vi "Get Monitor Variables.vi"(8 "error in (no error)":errorcluster, 9 "Channel":i32, 11 "LabVIEW Web Service Request":refnum<class "Web Request.lvclass">) -> (0 "error out":errorcluster, 3 "LabVIEW Web Service Request out":refnum<class "Web Request.lvclass">)   [LabVIEW 2018]
doc: "This VI sets all of the ESP variables for a single contact so it can be output from an ESP script."
uses:
  <vilib>/wsapi/Web Request.lvclass
  subvis/i32 to dec string small.vi
  CAEN globals.vi
  <vilib>/wsapi/class/subVIs/Set Many String ESP Variables.vi
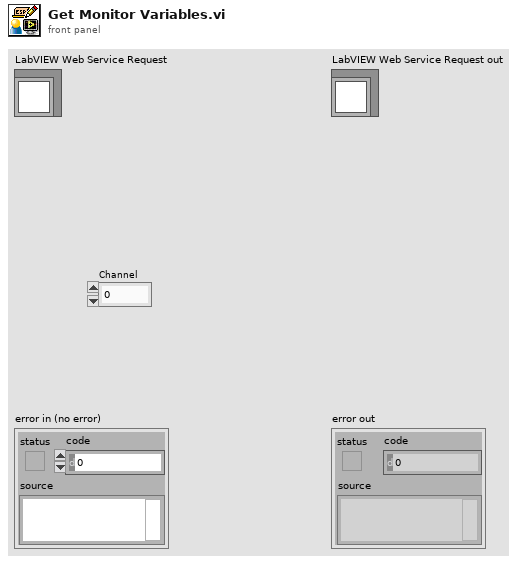
[diagram p1: front panel]
types:
  T1 = typedef "channel_cluster.ctl" = cluster{"Channel Name":string, "Crate":i32, "Card Type":string, "Card":i32, "Channel":i32, "Status Icon":picture, "Vmon (V)":dbl, "Vset (V)":dbl, "Imon (A)":dbl, "Iset (A)":dbl, "Timestamp":string, "ON/OFF":bool, "Status":string, "Vswmax (V)":dbl, "Flag":bool, "Vfile (V)":dbl, "Error Logged":bool[], "enable_file":bool}
  T2 = typedef "channel.ctl" = cluster{" Card.Channel":dbl, "Crate":i32}
  T3 = cluster{"Group Name":string, "Channels in Group":T2[]}[]
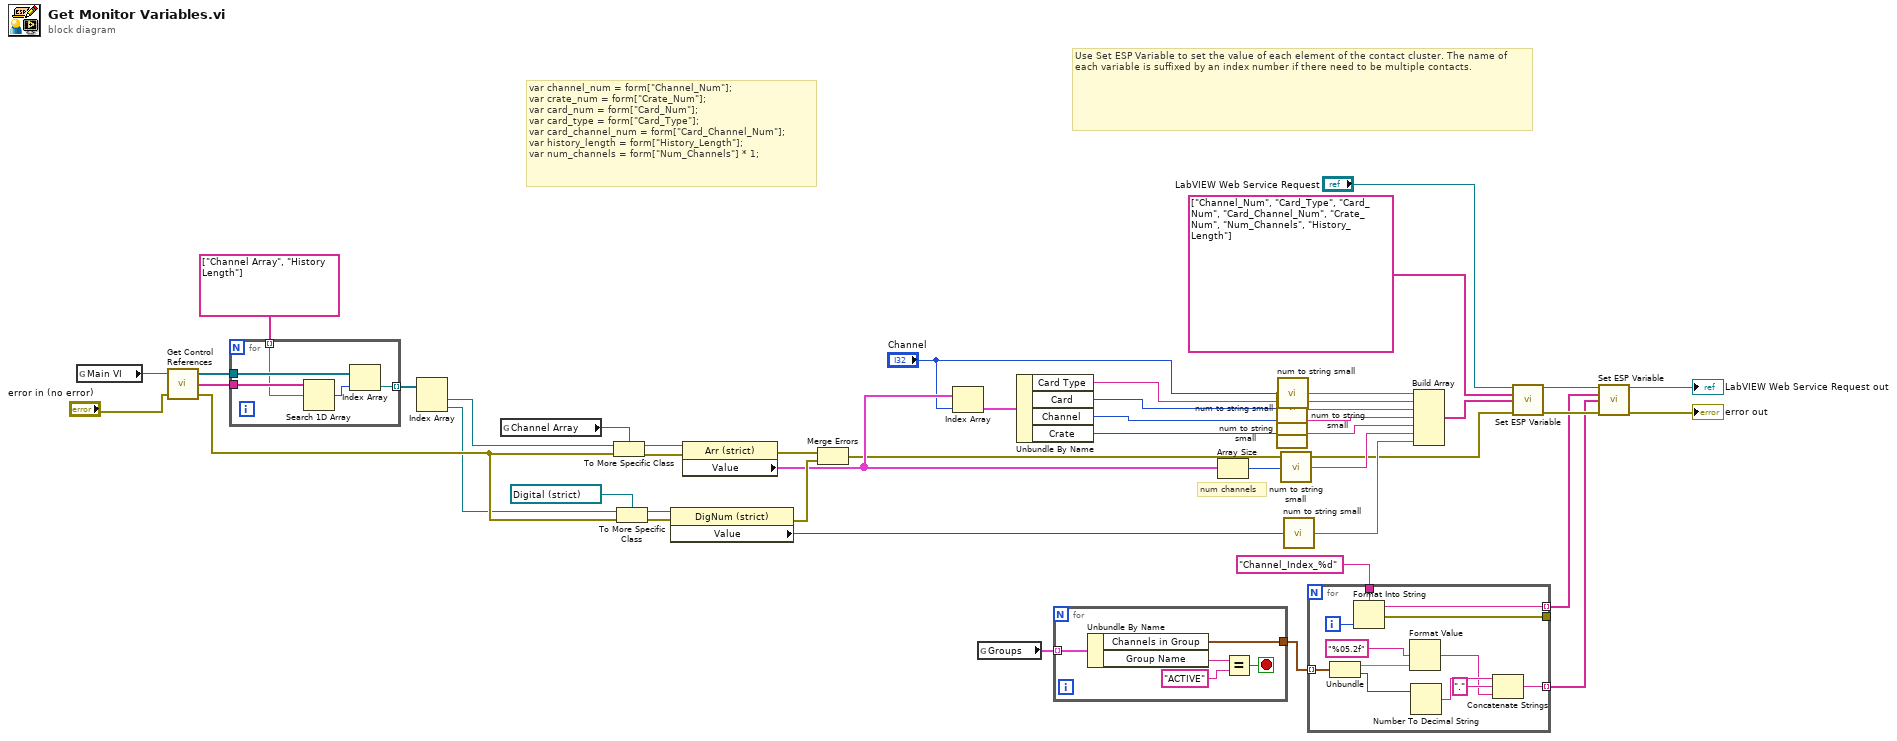
[diagram p0: block diagram]
diagram:
  # "var channel_num = form[\"Channel_Num\"]; \nvar crate_num = form[\"Crate_Num\"];\nvar card_num = form[\"Card_Num\"];\nvar card_type = form[\"Card_Type\"];\nvar card_channel_num = form[\"Card_Channel_Num\"];\nvar history_length = form[\"History_Length\"];\nvar num_channels = form[\"Num_Channels\"] * 1;"
  # "num channels"
  # "Use Set ESP Variable to set the value of each element of the contact cluster. The name of each variable is suffixed by an index number if there need to be multiple contacts."
  n1 = global read "CAEN globals.vi" "Main VI"() -> (w45:refnum<vi>)
  n2 = call "Get Control References.vi"("error in"="error in (no error)", "This vi"=w45) -> ("error out"=w27:errorcluster, "Control Names"=w44:string[], "Controls[]"=w43:refnum<vi>[])  [unwired: 1 in]
  n3 = for {
    tunnel: w44 -> [w50]
    tunnel: w43 -> [w48]
    tunnel: [w47] -> w41 mode=indexing
    tunnel: string[] ["Channel Array", "History Length"] ("Control Names") -> [w46] mode=indexing
    n4 = Search 1D Array(1D array=w50, element=w46) -> (index of element=w49:i32)  [unwired: 1 in]
    n5 = Index Array(array=w48, index=w49) -> (element=w47:refnum<vi>)
  }
  n6 = Index Array(array=w41) -> (element #1=w38:refnum<vi>, element #2=w25:refnum<vi>)  [unwired: 2 in]
  n7 = global read "CAEN globals.vi" "Channel Array"() -> (w3:refnum<vi>)
  n8 = To More Specific Class(target class=w3, reference=w38, error in=w27) -> (specific class reference=w40:refnum<vi>, error out=w39:errorcluster)
  n9 = To More Specific Class(target class=refnum<vi> refnum ("History Length"), reference=w25, error in=w27) -> (specific class reference=w29:refnum<vi>, error out=w26:errorcluster)
  n10 = property class="DigNum (strict)"(reference=w29, error in=w26) -> (error out=w24:errorcluster, "Value"=w23:i32)  [unwired: 1 out]
  n11 = property class="Arr (strict)"(reference=w40, error in=w39) -> (error out=w19:errorcluster, "Value"=w18:T1[])  [unwired: 1 out]
  n12 = Merge Errors(w19, w24) -> (w16:errorcluster)
  n13 = Index Array(array=w18, index="Channel") -> (element=w17:T1)
  n14 = global read "CAEN globals.vi" "Groups"() -> (w6:T3)
  n15 = Unbundle By Name(w17) -> ("Card Type"=w15:string, "Card"=w14:i32, "Channel"=w13:i32, "Crate"=w12:i32)
  n16 = for {
    tunnel: w6 -> [w52] mode=indexing
    tunnel: [w51] -> w2
    stop <- w53 stop-if-true
    n17 = Unbundle By Name(w52) -> ("Channels in Group"=w51:T2[], "Group Name"=w55:string)
    n18 = Equal?(x=w55, y="ACTIVE") -> (x = y?=w53:bool)
  }
  n19 = Array Size(array=w18) -> (size(s)=w37:i32)
  n20 = call-poly "num to string small.vi"("number"=w14) -> ("String"=w35:string)  [unwired: 14 in]
  n21 = call-poly "num to string small.vi"("number"=w13) -> ("String"=w34:string)  [unwired: 14 in]
  n22 = call-poly "num to string small.vi"("number"=w12) -> ("String"=w33:string)  [unwired: 14 in]
  n23 = call-poly "num to string small.vi"("number"="Channel") -> ("String"=w36:string)  [unwired: 14 in]
  n24 = call-poly "num to string small.vi"("number"=w37) -> ("String"=w32:string)  [unwired: 14 in]
  n25 = call-poly "num to string small.vi"("number"=w23) -> ("String"=w22:string)  [unwired: 14 in]
  n26 = for {
    tunnel: w2 -> [w63] mode=indexing
    tunnel: [w66] -> _
    tunnel: "Channel_Index_%d" ("y") -> [w65]
    tunnel: [w64] -> w4 mode=indexing
    tunnel: [w58] -> w1 mode=indexing
    i -> [w67]
    n27 = Unbundle(w63) -> ("Card.Channel"=w57:dbl, "Crate"=w62:i32)
    n28 = Format Into String(format string=w65, w67) -> (resulting string=w64:string, error out=w66:errorcluster)  [unwired: 2 in]
    n29 = Format Value(format string="%05.2f" ("y"), value (0)=w57) -> (output string=w59:string)  [unwired: 1 in]
    n30 = Number To Decimal String(number=w62) -> (decimal integer string=w61:string)  [unwired: 1 in]
    n31 = Concatenate Strings(w61, "." ("string"), w59) -> (w58:string)
  }
  n32 = Build Array(w36, w15, w35, w34, w33, w32, w22) -> (w30:string[])
  n33 = call-poly <vilib>:"Set ESP Variable.vi"("LabVIEW Web Service Request"="LabVIEW Web Service Request", "keys"=string[] ["Channel_Num", "Card_Type", "Card_Num", "Card_Channel_Num", "Crate_Num", "Num_Channels", "History_Length"] ("appended array"), "values"=w30, "error in (no error)"=w16) -> ("LabVIEW Web Service Request out"=w9:refnum<class "Web Request.lvclass">, "error out"=w10:errorcluster)  [unwired: 10 in]
  n34 = call-poly <vilib>:"Set ESP Variable.vi"("LabVIEW Web Service Request"=w9, "keys"=w4, "values"=w1, "error in (no error)"=w10) -> ("LabVIEW Web Service Request out"=→"LabVIEW Web Service Request out":refnum<class "Web Request.lvclass">, "error out"=→"error out":errorcluster)  [unwired: 10 in]
